vi "ASI_Init.vi"() -> (1 "Status":bool, 2 "Positions":dbl[](array[numeric]), 3 "VISA Refnum out":refnum<visa-resource-name>)   [LabVIEW 2014]
uses:
  <vilib>/Instr/_visa.llb/VISA Configure Serial Port (Instr).vi
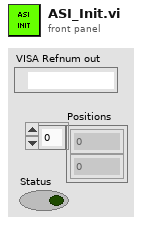
[diagram p1: front panel]
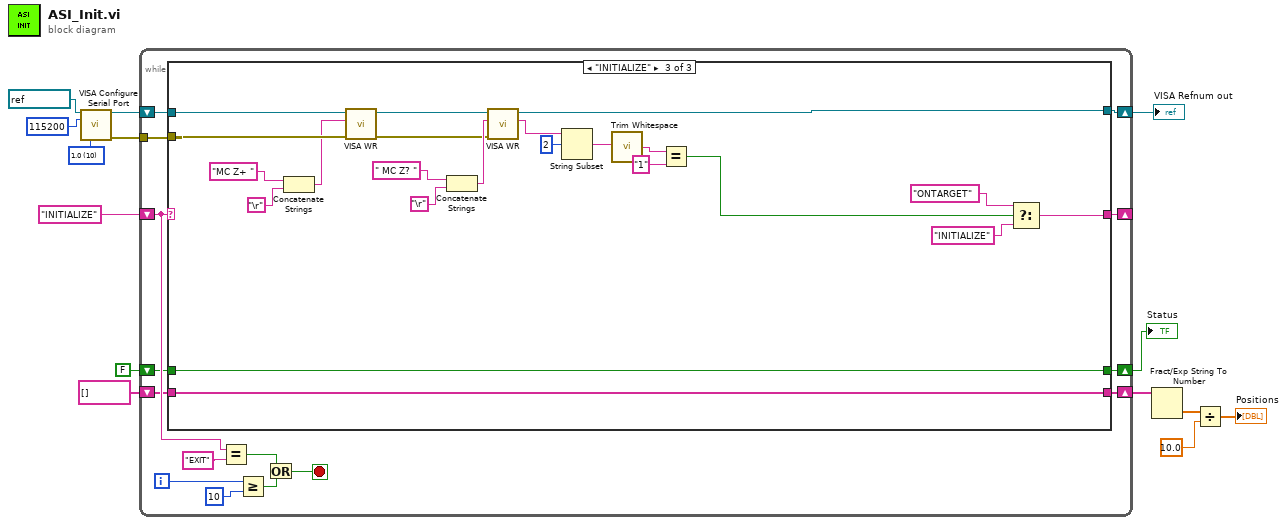
[diagram p0: block diagram]
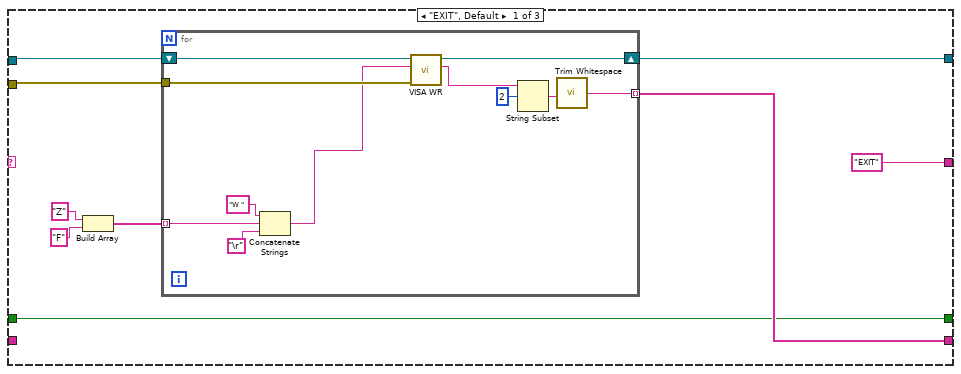
[diagram p2: hidden frame]
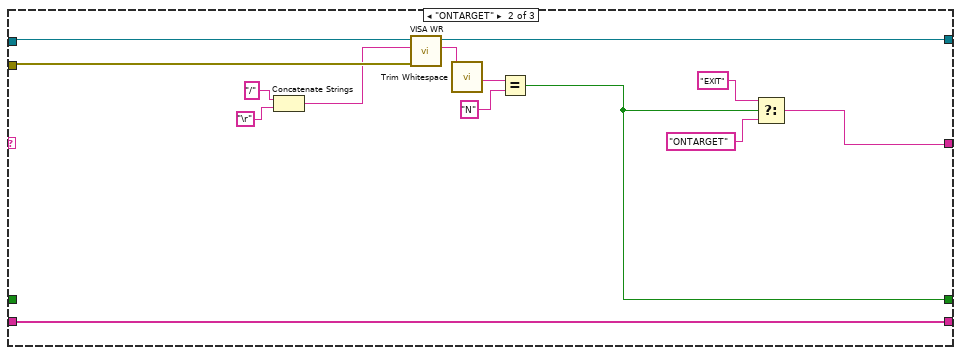
[diagram p3: hidden frame]
diagram:
  w10 = u16 10 items=["1.0"=10, "1.5"=15, "2.0"=20] ("stop bits (10: 1 bit)")
  n1 = call-poly "VISA Configure Serial Port"("VISA resource name"=refnum<visa-resource-name> "COM8", "baud rate (9600)"=u32 115200, "stop bits (10: 1 bit)"=w10) -> ("VISA resource name out"=w14:refnum<visa-resource-name>, "error out"=w11:errorcluster)  [unwired: 11 in]
  n2 = while {
    tunnel: w11 -> [w28]
    shift-right: [w27] -> _
    shift-left: "INITIALIZE" -> [w25]
    shift-right: [w17] -> w7
    shift-left: w14 -> [w29]
    shift-right: [w18] -> w4
    shift-left: string[] [] -> [w16]
    shift-right: [w21] -> w13
    shift-left: FALSE -> [w15]
    i -> [w19]
    stop <- w23 stop-if-true
    n3 = case shown="\"INITIALIZE\"" w25 {
      tunnel: w29 -> [w37 w63 w85]
      tunnel: w28 -> [w36 w62 w76]
      tunnel: [w33 w50 w64] -> w21
      tunnel: ["EXIT" w57 w66] -> w27
      tunnel: [w35 w56 w81] -> w18
      tunnel: [w34 w60 w80] -> w17
      tunnel: w16 -> [_ w56 w81]
      tunnel: w15 -> [w33 _ w64]
      frame "EXIT", Default {
        n4 = Build Array("Z", "F") -> (w30:string[])
        n5 = for {
          tunnel: w36 -> [w48]
          tunnel: [w45] -> w35 mode=indexing
          tunnel: w30 -> [w43] mode=indexing
          shift-right: [w44] -> w34
          shift-left: w37 -> [w49]
          n6 = Concatenate Strings("W " ("string"), w43, "\r") -> (w47:string)
          n7 = call "VISA WR.vi"("error in (no error)"=w48, "write buffer"=w47, "VISA Refnum in"=w49) -> ("read buffer"=w46:string, "VISA Refnum out"=w44:refnum<visa-resource-name>)  [unwired: 6 in, 1 out]
          n8 = String Subset(string=w46, offset (0)=2) -> (substring=w39:string)  [unwired: 1 in]
          n9 = call <vilib>:"Trim Whitespace.vi"("string"=w39) -> ("trimmed string"=w45:string)  [unwired: 1 in]
        }
      }
      frame "ONTARGET" {
        n10 = Concatenate Strings("/" ("string"), "\r") -> (w61:string)
        n11 = call "VISA WR.vi"("error in (no error)"=w62, "write buffer"=w61, "VISA Refnum in"=w63) -> ("read buffer"=w53:string, "VISA Refnum out"=w60:refnum<visa-resource-name>)  [unwired: 6 in, 1 out]
        n12 = call <vilib>:"Trim Whitespace.vi"("string"=w53) -> ("trimmed string"=w51:string)  [unwired: 1 in]
        n13 = Equal?(x=w51, y="N") -> (x = y?=w50:bool)
        n14 = Select(t="EXIT", s=w50, f="ONTARGET") -> (s? t:f=w57:string)
      }
      frame "INITIALIZE" {
        n15 = Concatenate Strings("MC Z+ " ("string"), "\r") -> (w72:string)
        n16 = call "VISA WR.vi"("error in (no error)"=w76, "write buffer"=w72, "VISA Refnum in"=w85) -> ("error out"=w75:errorcluster, "VISA Refnum out"=w77:refnum<visa-resource-name>)  [unwired: 6 in, 1 out]
        n17 = Concatenate Strings(" MC Z? " ("string"), "\r") -> (w84:string)
        n18 = call "VISA WR.vi"("error in (no error)"=w75, "write buffer"=w84, "VISA Refnum in"=w77) -> ("read buffer"=w71:string, "VISA Refnum out"=w80:refnum<visa-resource-name>)  [unwired: 6 in, 1 out]
        n19 = String Subset(string=w71, offset (0)=2) -> (substring=w69:string)  [unwired: 1 in]
        n20 = call <vilib>:"Trim Whitespace.vi"("string"=w69) -> ("trimmed string"=w68:string)  [unwired: 1 in]
        n21 = Equal?(x=w68, y="1") -> (x = y?=w65:bool)
        n22 = Select(t="ONTARGET", s=w65, f="INITIALIZE") -> (s? t:f=w66:string)
      }
    }
    n23 = Equal?(x=w25, y="EXIT") -> (x = y?=w24:bool)
    n24 = Greater Or Equal?(x=w19, y=10 ("x")) -> (x >= y?=w22:bool)
    n25 = Or(x=w24, y=w22) -> (x .or. y?=w23:bool)
  }
  "VISA Refnum out" <- w7
  "Status" <- w13
  n26 = Fract/Exp String To Number(string=w4) -> (number=w2:dbl[])  [unwired: 3 in, 1 out]
  n27 = Divide(x=w2, y=10.0) -> (x/y=→"Positions":dbl[])
